vi "Set Pump State.vi"(8 "error in (no error)":cluster{"状态":bool, "代码":i32, "源":string} caption="错误输入（无错误）", 10 "泵状态":bool, 11 "蒸发冷却器输入":refnum<class "Evaporative Cooler.lvclass">) -> (0 "error out":cluster{"状态":bool, "代码":i32, "源":string} caption="错误输出")   [LabVIEW 2013, in "Evaporative Cooler.lvlib" / "Evaporative Cooler.lvclass"]
doc: "子类中必须对该方法进行重写以按输入参数值开关水泵。"
uses:
  Evaporative Cooler.lvclass
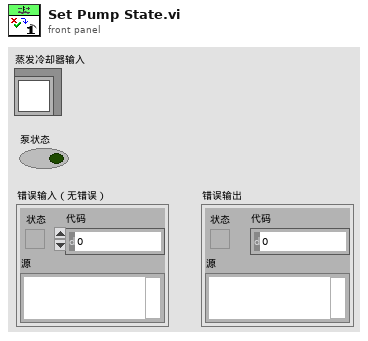
[diagram p1: front panel]
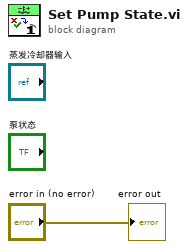
[diagram p0: block diagram]
diagram:
  "error out" <- "error in (no error)"
